vi "Create Command.vi"(8 "error in (no error)":errorcluster caption="错误输入（无错误）", 10 "cmdText":string, 11 "OleDBClass 输入":refnum<class "OleDBClass.lvclass"> caption="DNL_LabVIEW Object in") -> (0 "error out":errorcluster caption="错误输出", 3 "OleDBClass 输出":refnum<class "OleDBClass.lvclass"> caption="DNL_LabVIEW Object out")   [LabVIEW 2012, in "OleDBClass.lvclass"]
uses:
  OleDBClass.lvclass
  OleDBClass.lvclass/OleDBClass.ctl
  System.Data
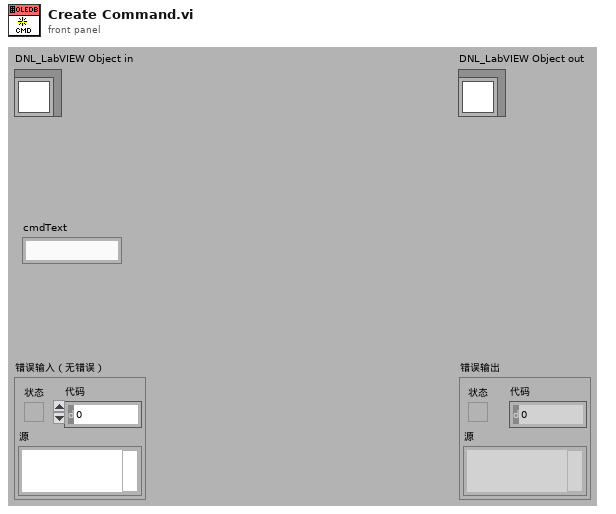
[diagram p1: front panel]
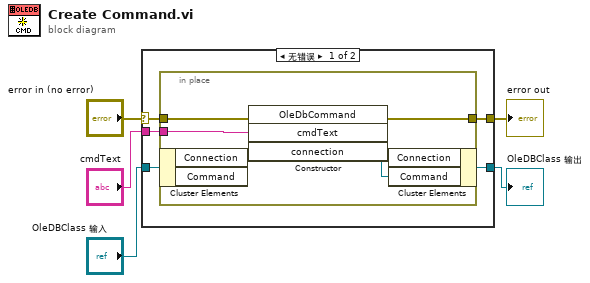
[diagram p0: block diagram]
diagram:
  n1 = case shown="无错误" "error in (no error)" {
    selector: "error in (no error)" -> [w9 w17]
    tunnel: [w6 w17] -> w4
    tunnel: [w7 w16] -> w2
    tunnel: "OleDBClass 输入" -> [w10 w16]
    tunnel: "cmdText" -> [w8 _]
    frame No Error {
      n2 = in-place {
        in-place-border: w9 -> [w15]
        in-place-border: w8 -> [w14]
        in-place-border: [w11] -> w6
        n3 = in-place-cluster #1(w10) -> ("Connection"=w12:refnum<k24>)  [unwired: 1 out]
        n4 = constructor class="OleDbCommand"(error in=w15, "cmdText"=w14, "connection"=w12) -> (reference out=w13:refnum<k24>, error out=w11:errorcluster)  [unwired: 2 in, 3 out]
        n5 = in-place-cluster #1("Connection"=w12, "Command"=w13) -> (w7:refnum<class "OleDBClass.lvclass">)
      }
    }
    frame Error {
    }
  }
  "error out" <- w4
  "OleDBClass 输出" <- w2
